vi "Square and Add.vi"(5 "Real":fxp<+/-,16,1> format="%.16g", 7 "Imaginary":fxp<+/-,16,1> format="%.16g") -> (6 "Magnitude^2":fxp<+/-,30,3> format="%.28g")   [LabVIEW 2011]
uses:
  <vilib>/rvi/FXPMathLib/basic elements/DSP48E/simVIs/niFpgaDsp48eRegisters.ctl
  <vilib>/rvi/FXPMathLib/basic elements/DSP48E/simVIs/niFpgaDsp48eEnables.ctl
  <vilib>/rvi/FXPMathLib/basic elements/DSP48E/simVIs/niFpgaDsp48eResets.ctl
  <vilib>/rvi/FXPMathLib/basic elements/DSP48E/simVIs/niFpgaDsp48eSimulationState.ctl
  <vilib>/rvi/FXPMathLib/basic elements/DSP48E/subVIs/niFpgaDsp48eType.ctl
  <vilib>/rvi/FXPMathLib/basic elements/DSP48E/subVIs/niFpgaDsp48eAlumodeOpmodeCarryinselState.ctl
  <vilib>/rvi/FXPMathLib/basic elements/DSP48E/subVIs/niFpgaDsp48eUseMultiplierState.ctl
  <vilib>/rvi/FXPMathLib/basic elements/DSP48E/subVIs/niFpgaDsp48eLogicUnitModeState.ctl
  <vilib>/rvi/FXPMathLib/basic elements/DSP48E/subVIs/niFpgaDsp48eSelectPatternState.ctl
  <vilib>/rvi/FXPMathLib/basic elements/DSP48E/subVIs/niFpgaDsp48eSelectMaskState.ctl
  <vilib>/rvi/FXPMathLib/basic elements/DSP48E/subVIs/niFpgaDsp48eAutoresetState.ctl
  <vilib>/rvi/FXPMathLib/basic elements/DSP48E/simVIs/niFpgaDsp48eSimMultiplier.vi
  <vilib>/rvi/FXPMathLib/basic elements/DSP48E/simVIs/niFpgaDsp48eSimArithmetic.vi
  <vilib>/rvi/FXPMathLib/basic elements/DSP48E/simVIs/niFpgaDsp48eSimPatternDetect.vi
  <vilib>/rvi/FXPMathLib/basic elements/DSP48E/simVIs/niFpgaDsp48eSimP.vi
  <vilib>/rvi/FXPMathLib/basic elements/DSP48E/simVIs/niFpgaDsp48eSimUpdateState.vi
  <vilib>/rvi/FXPMathLib/basic elements/DSP48E/simVIs/niFpgaDsp48eCheckMode.vi
  <vilib>/rvi/FXPMathLib/basic elements/DSP48E/simVIs/niFpgaDsp48eReportInvalidMode.vi
  <vilib>/rvi/FXPMathLib/FxpInterpret/XNode/nifxpmath_Interpret.xnode
  <vilib>/rvi/FXPMathLib/basic elements/DSP48E/XNode/niFpgaDsp48e.xnode
panel:
  out "fixed-point":fxp<+/-,30,1> format="%.30g"
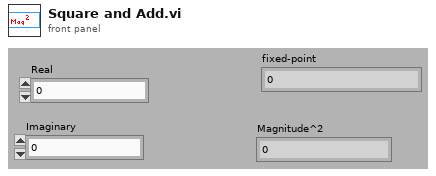
[diagram p1: front panel]
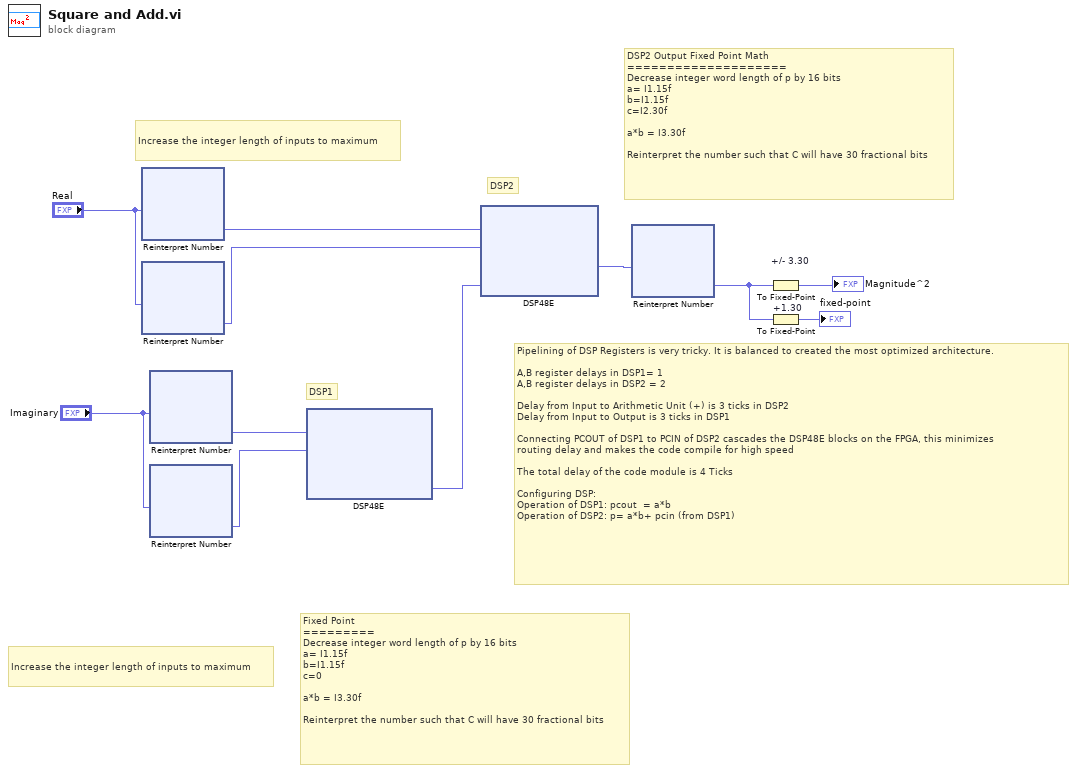
[diagram p0: block diagram]
diagram:
  # "Increase the integer length of inputs to maximum"
  # "DSP2"
  # "DSP1"
  # "Pipelining of DSP Registers is very tricky. It is balanced to created the most optimized architecture.\n\nA,B register delays in DSP1= 1\nA,B register delays in DSP2 = 2\n\nDelay from Input to Arithmetic Unit (+) is 3 ticks in DSP2\nDelay from Input to Output is 3 ticks in DSP1\n\nConnecting PCOUT of DSP1 to PCIN of DSP2 cascades the DSP48E blocks on the FPGA, this minimizes\nrouting delay and makes the code compile for high speed\n\nThe total delay of the code module is 4 Ticks\n\nConfiguring DSP:\nOperation of DSP1: pcout  = a*b\nOperation of DSP2: p= a*b+ pcin (from DSP1)"
  # "DSP2 Output Fixed Point Math\n====================\nDecrease integer word length of p by 16 bits\na= I1.15f\nb=I1.15f\nc=I2.30f\n\na*b = I3.30f\n\nReinterpret the number such that C will have 30 fractional bits"
  # "Increase the integer length of inputs to maximum"
  # "Fixed Point\n=========\nDecrease integer word length of p by 16 bits\na= I1.15f\nb=I1.15f\nc=0\n\na*b = I3.30f\n\nReinterpret the number such that C will have 30 fractional bits"
  n1 = xnode "Reinterpret Number"("x"="Real") -> ("y"=w6:fxp<+/-,16,16>)
  n2 = xnode "Reinterpret Number"("x"="Real") -> ("y"=w7:fxp<+/-,16,16>)
  n3 = xnode "Reinterpret Number"("x"="Imaginary") -> ("y"=w11:fxp<+/-,16,16>)
  n4 = xnode "Reinterpret Number"("x"="Imaginary") -> ("y"=w10:fxp<+/-,16,16>)
  n5 = xnode "DSP48E"("a"=w11, "b"=w10) -> ("pcout"=w4:fxp<+/-,48,48>)  [unwired: 1 out]
  n6 = xnode "DSP48E"("a"=w6, "b"=w7, "pcin"=w4) -> ("p"=w5:fxp<+/-,48,48>)
  n7 = xnode "Reinterpret Number"("x"=w5) -> ("y"=w2:fxp<+/-,48,18>)
  n8 = To Fixed-Point "+/- 3.30"(number=w2) -> (fixed-point=→"Magnitude^2":fxp<+/-,30,3>)  [unwired: 1 in]
  n9 = To Fixed-Point "+1.30"(number=w2) -> (fixed-point=→"fixed-point":fxp<+/-,30,1>)  [unwired: 1 in]
